vi "playback test.vi"(5 "Rewind":bool, 6 "Record":bool, 7 "Playback":bool, 8 "Taper Limit":dbl=1.0, 9 "Playback allow":bool=TRUE, 10 "Encoder Recording Data":cluster{dbl, u32}[](array[cluster])=[{0.0, 40}, {5.5, 82}, {6.75, 122}, {7.0, 162}, {7.0, 203}, {7.25, 244}, {3.75, 283}, {2.5, 323}, {2.25, 363}, {-0.5, 403}, {-6.75, 444}, {-16.0, 485}, {-28.75, 525}, {-46.0, 565}, {-68.5, 607}, {-94.25, 647}, {-125.25, 689}, {-157.25, 730}, {-189.0, 770}, {-219.75, 811}, {-239.5, 851}, {-265.25, 892}, {-287.0, 932}, {-303.5, 973}, {-312.75, 1014}, {-315.0, 1055}, {-313.5, 1095}, {-306.25, 1136}, {-293.75, 1177}, {-277.0, 1219}, {-254.0, 1261}, {-227.25, 1302}, {-196.0, 1341}, {-158.5, 1382}, {-118.75, 1422}, {-76.75, 1463}, {-36.75, 1503}, {-3.0, 1543}, {26.0, 1583}, {56.5, 1625}, {81.75, 1665}, {100.5, 1706}, {112.5, 1746}, {116.75, 1787}, {116.75, 1828}, {113.0, 1868}, {105.0, 1909}, {92.75, 1949}, {76.25, 1990}, {55.25, 2030}, {29.5, 2071}, {-0.25, 2112}, {-35.25, 2152}, {-74.0, 2193}, {-116.25, 2233}, {-159.0, 2274}, {-202.75, 2314}, {-245.0, 2356}, {-274.5, 2396}, {-310.5, 2436}, {-341.5, 2477}, {-366.25, 2517}, {-383.0, 2558}, {-390.25, 2599}, {-390.75, 2640}, {-387.0, 2681}, {-378.0, 2722}, {-363.0, 2763}, {-343.5, 2804}, {-318.25, 2845}, {-287.0, 2885}, {-248.75, 2926}, {-205.0, 2967}, {-155.75, 3008}, {-102.25, 3049}, {-50.5, 3088}, {1.0, 3130}, {41.25, 3171}, {84.0, 3212}, {122.0, 3253}, {153.75, 3294}, {180.5, 3335}, {200.25, 3375}, {213.5, 3416}, {218.25, 3457}, {218.25, 3496}, {213.5, 3536}, {205.0, 3576}, {192.0, 3617}, {175.0, 3658}, {152.25, 3699}, {125.25, 3740}, {93.5, 3781}, {56.0, 3822}, {13.75, 3863}, {-31.25, 3903}, {-80.25, 3944}, {-130.5, 3986}, {-177.75, 4027}, {-214.25, 4068}, {-253.75, 4108}, {-291.5, 4149}, {-326.0, 4190}, {-356.75, 4231}, {-384.75, 4272}, {-409.5, 4313}, {-431.0, 4353}, {-449.5, 4393}, {-466.0, 4433}, {-479.5, 4474}, {-491.0, 4515}, {-500.0, 4556}, {-506.5, 4597}, {-510.75, 4636}, {-513.0, 4678}, {-513.5, 4718}, {-513.5, 4758}, {-513.5, 4800}, {-513.5, 4840}, {-513.5, 4882}, {-513.5, 4923}, {-513.5, 4964}, {-513.5, 5005}, {-513.5, 5045}, {-513.5, 5085}, {-513.5, 5127}, {-513.5, 5168}, {-513.5, 5211}, {-513.5, 5250}, {-513.5, 5291}, {-513.5, 5331}, {-513.5, 5372}, {-513.5, 5413}, {-513.5, 5454}], 11 "Hardware In":T5={"Motor Selection"="Test motor thing", "EncoderDevRef"={"DevStatus"={"status"=FALSE, "code"=0, "source"=""}, "EncoderIndex"=enum."Enc 0", "CounterIndex"=enum."Invalid", "DistancePerCount"=1.0, "Decoding Type"=enum."4x"}}) -> (0 "Encoder Distance PB":dbl)   [LabVIEW 2017]
uses:
  <vilib>/addons/control/pid/NI_PID_pid.lvlib
  <vilib>/addons/control/pid/pid.llb/PID (DBL).vi
  <vilib>/Rock Robotics/WPI/RobotDrive/WPI_RobotDriveArcadeDrive_Standard(NoSaturation).vi
  <vilib>/Rock Robotics/SystemInterfaces/Encoder/FPGA_EncoderIdx.ctl
  <vilib>/Rock Robotics/WPI/Encoder/WPI_EncoderType.ctl
  <vilib>/Rock Robotics/SystemInterfaces/Counter/FPGA_CounterCtrSystemIndex.ctl
  <vilib>/Rock Robotics/WPI/Encoder/WPI_EncoderDevRef.ctl
panel:
  out "Waveform Chart":cluster{dbl, dbl}(graph)
  in  "Playback PID gains":T6={"proportional gain (Kc)"=0.004, "integral time (Ti, min)"=0.0, "derivative time (Td, min)"=0.0} {"derivative time (Td, min)" format="%.8f"; "integral time (Ti, min)" format="%.8f"; "proportional gain (Kc)" format="%.8f"}
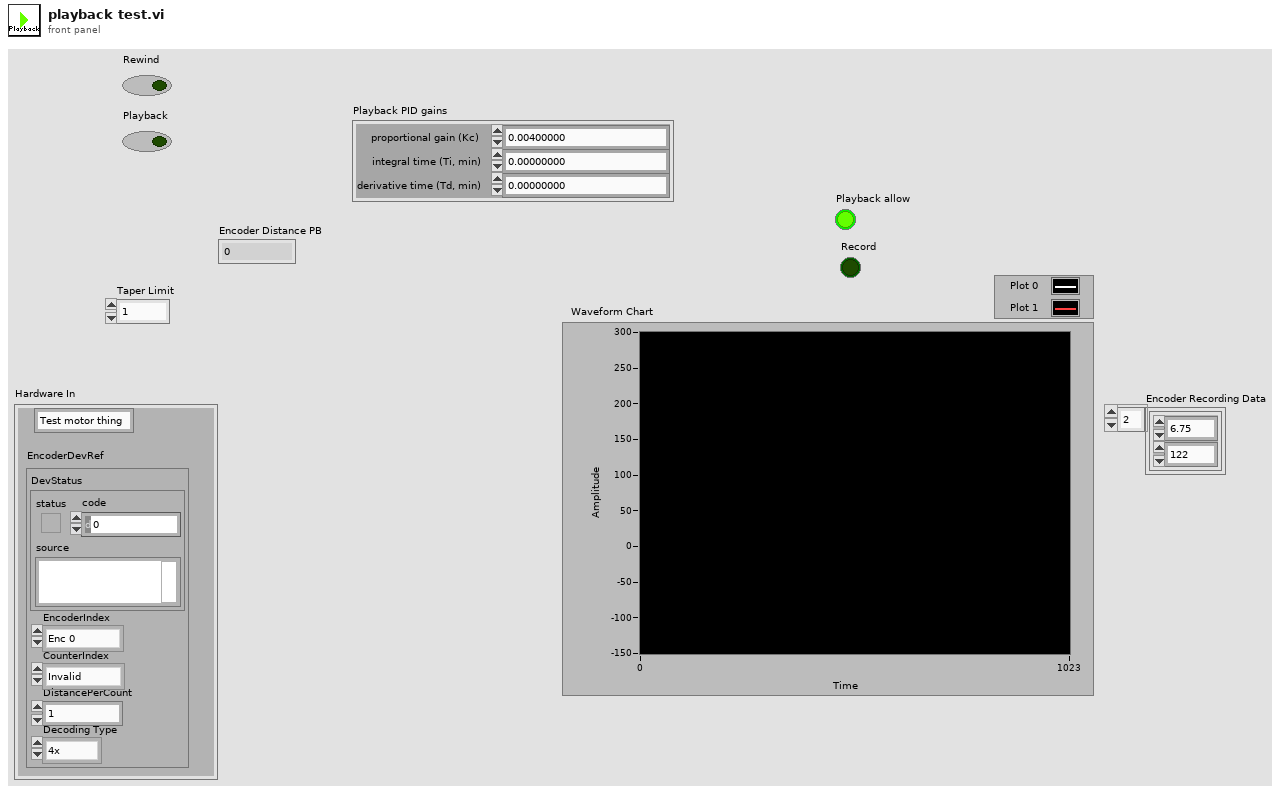
[diagram p1: front panel]
types:
  T1 = typedef "WPI_EncoderDevRef.ctl" = cluster{"DevStatus":errorcluster, "EncoderIndex":T2, "CounterIndex":T3, "DistancePerCount":dbl, "Decoding Type":T4}
  T2 = typedef "FPGA_EncoderIdx.ctl" = enum8{"Enc 0", "Enc 1", "Enc 2", "Enc 3", "Enc 4", "Enc 5", "Enc 6", "Enc 7", "Invalid"}
  T3 = typedef "FPGA_CounterCtrSystemIndex.ctl" = enum8{"Ctr 0", "Ctr 1", "Ctr 2", "Ctr 3", "Ctr 4", "Ctr 5", "Ctr 6", "Ctr 7", "Invalid"}
  T4 = typedef "WPI_EncoderType.ctl" = enum16{"1x", "2x", "4x"}
  T5 = cluster{"Motor Selection":string, "EncoderDevRef":T1}
  T6 = cluster{"proportional gain (Kc)":dbl, "integral time (Ti, min)":dbl, "derivative time (Td, min)":dbl}
  T7 = typedef "WPI_RobotDriveDevRef.ctl" = cluster{"DevStatus":errorcluster, "Motors[]":T8[], "Square Inputs":bool, "Max Output":dbl}
  T8 = typedef "WPI_MotorControlDeviceRef.ctl" = cluster{"DeviceStatus":errorcluster, "Type":T9, "PWM":cluster{"PWM Channel":T10, "DeadBand":T11}, "CAN":cluster{"Device Number":u8, "SetOutput VI Ref":variant, "GetOutput VI Ref":variant, "Enable VI Ref":variant, "Disable VI Ref":variant, "Data":variant}, "Invert":bool, "DIO PWM":cluster{"PWM \"Enable\" Channel":T10, "DIOChannel":T12, "PWM Rate":dbl}}
  T9 = typedef "WPI_MotorControlType.ctl" = enum16{"PWM", "CAN", "DIO PWM"}
  T10 = typedef "FPGA_DIOPWMChannel.ctl" = enum8{"PWM 0", "PWM 1", "PWM 2", "PWM 3", "PWM 4", "PWM 5", "PWM 6", "PWM 7", "PWM 8", "PWM 9", "PWM MXP 0", "PWM MXP 1", "PWM MXP 2", "PWM MXP 3", "PWM MXP 4", "PWM MXP 5", "PWM MXP 6", "PWM MXP 7", "PWM MXP 8", "PWM MXP 9", "Invalid"}
  T11 = typedef "WPI_PWMDeadband.ctl" = cluster{"Name":string, "maxPositivePwm":i32, "minPositivePwm":i32, "centerPwm":i32, "maxNegativePwm":i32, "minNegativePwm":i32, "angularRange":u16}
  T12 = typedef "FPGA_DIOChannel.ctl" = enum8{"DIO 0", "DIO 1", "DIO 2", "DIO 3", "DIO 4", "DIO 5", "DIO 6", "DIO 7", "DIO 8", "DIO 9", "DIO MXP 0", "DIO MXP 1", "DIO MXP 2", "DIO MXP 3", "DIO MXP 4", "DIO MXP 5", "DIO MXP 6", "DIO MXP 7", "DIO MXP 8", "DIO MXP 9", "DIO MXP 10", "DIO MXP 11", "DIO MXP 12", "DIO MXP 13", "DIO MXP 14", "DIO MXP 15", "SPI Port CS1", "SPI Port CS2", "SPI Port CS3", "SPI Port MISO", "SPI Port MOSI", "Invalid"}
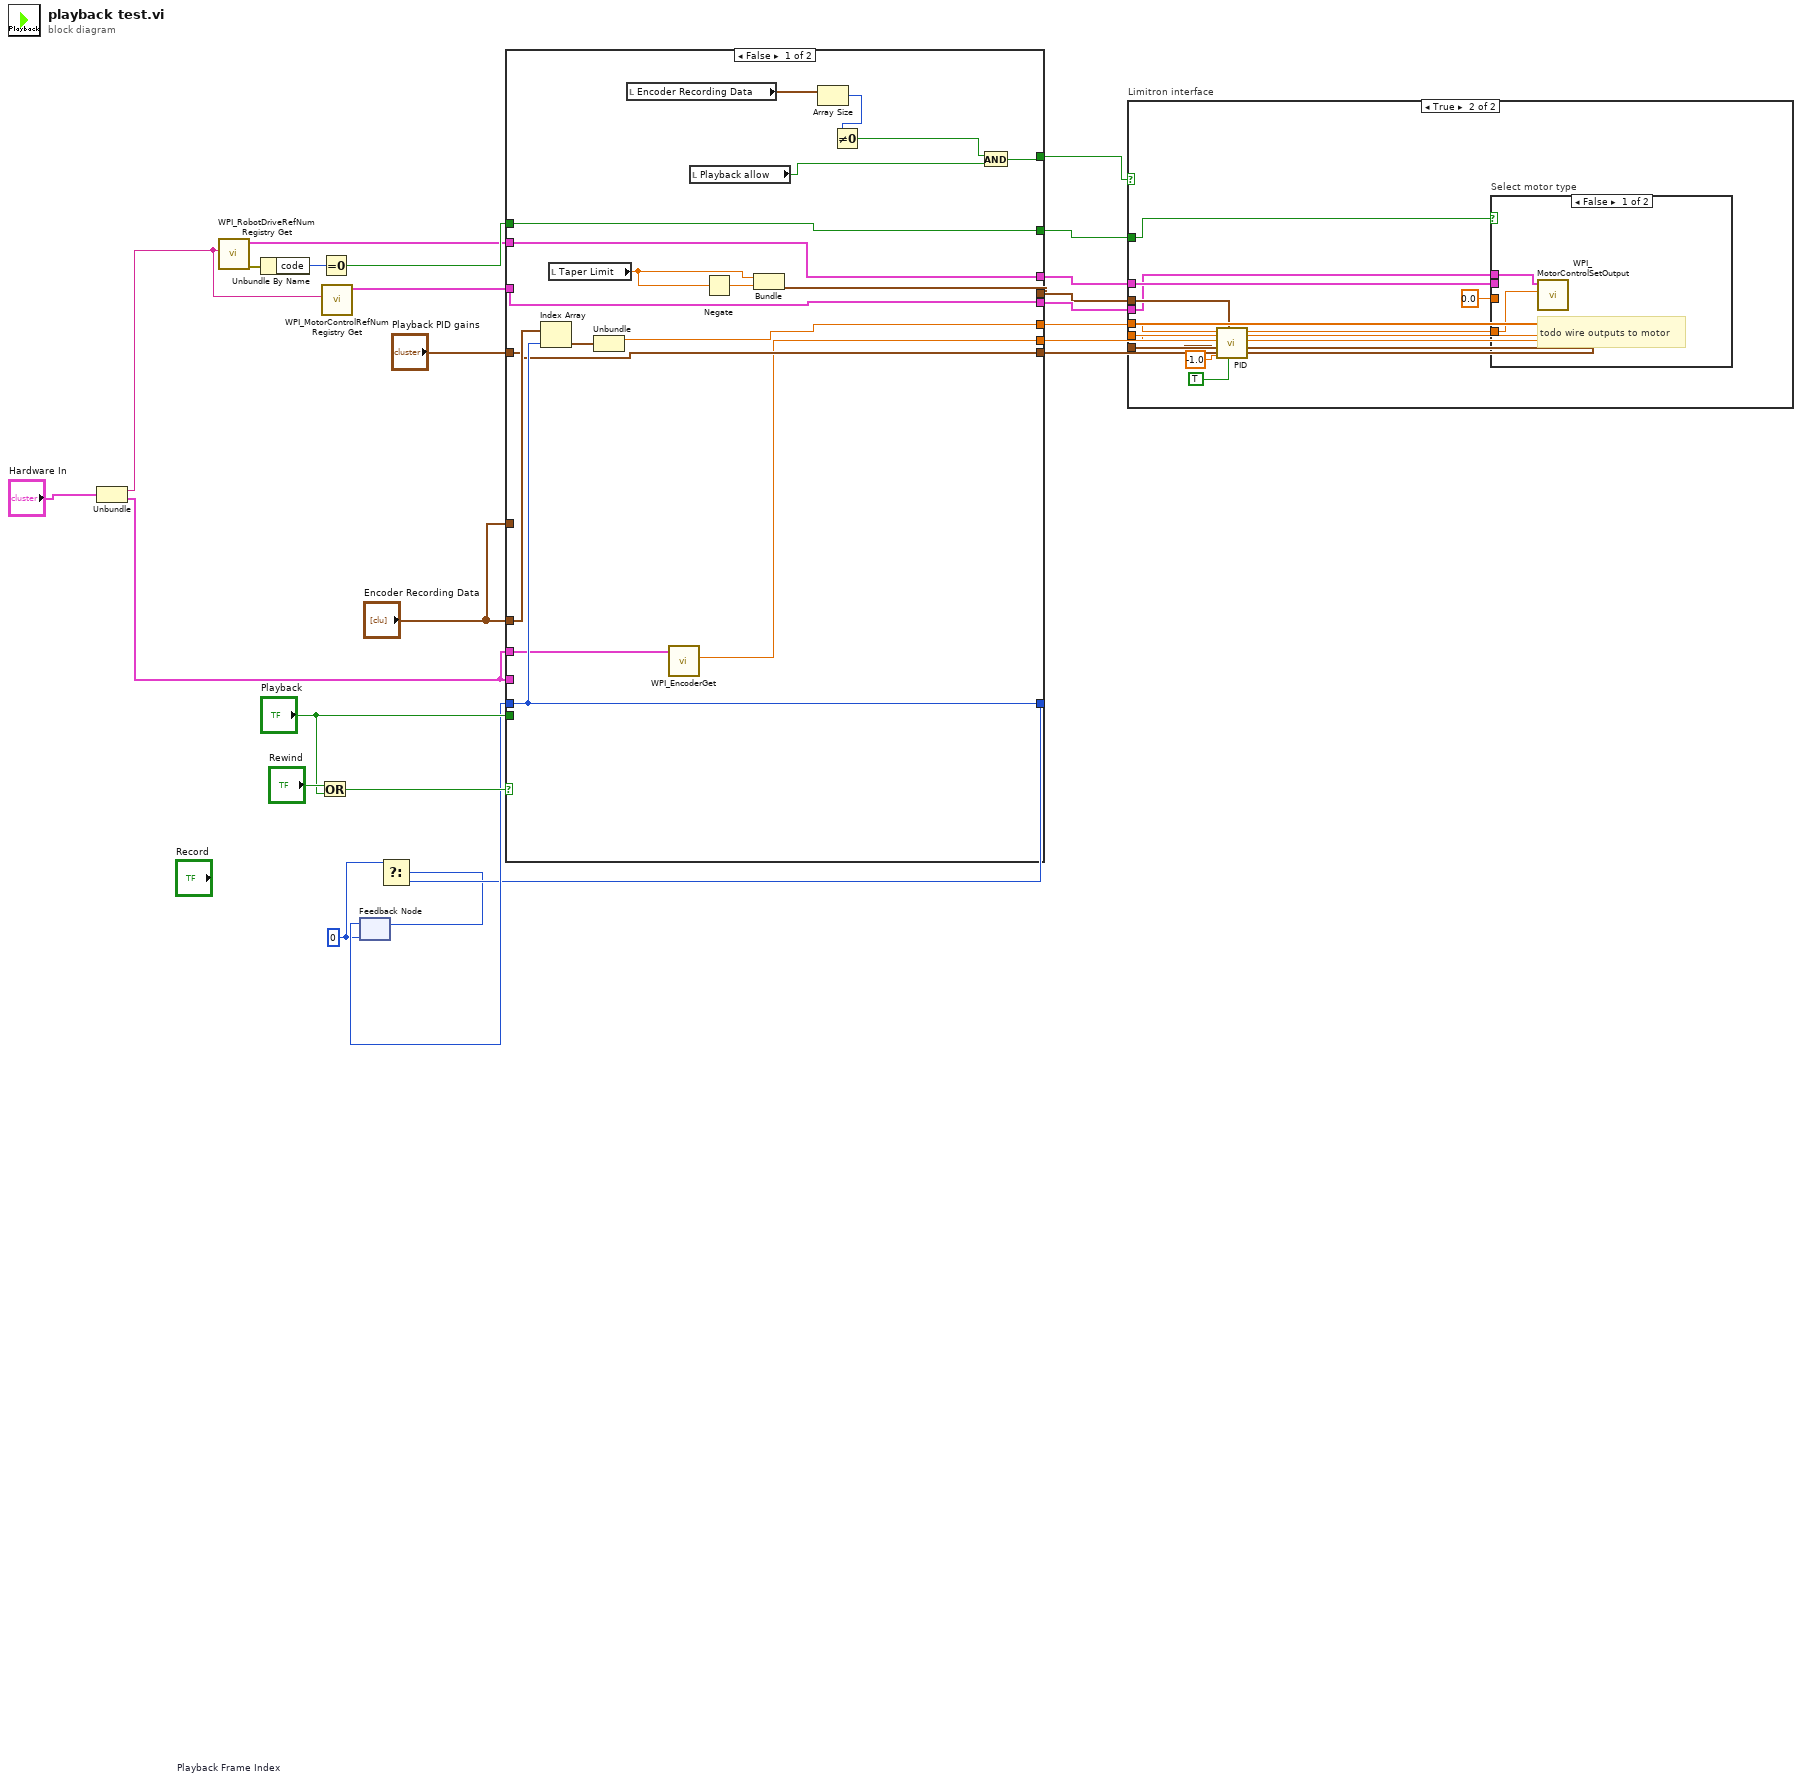
[diagram p0: block diagram]
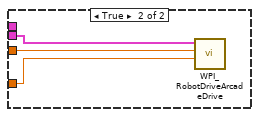
[diagram p3: hidden frame]
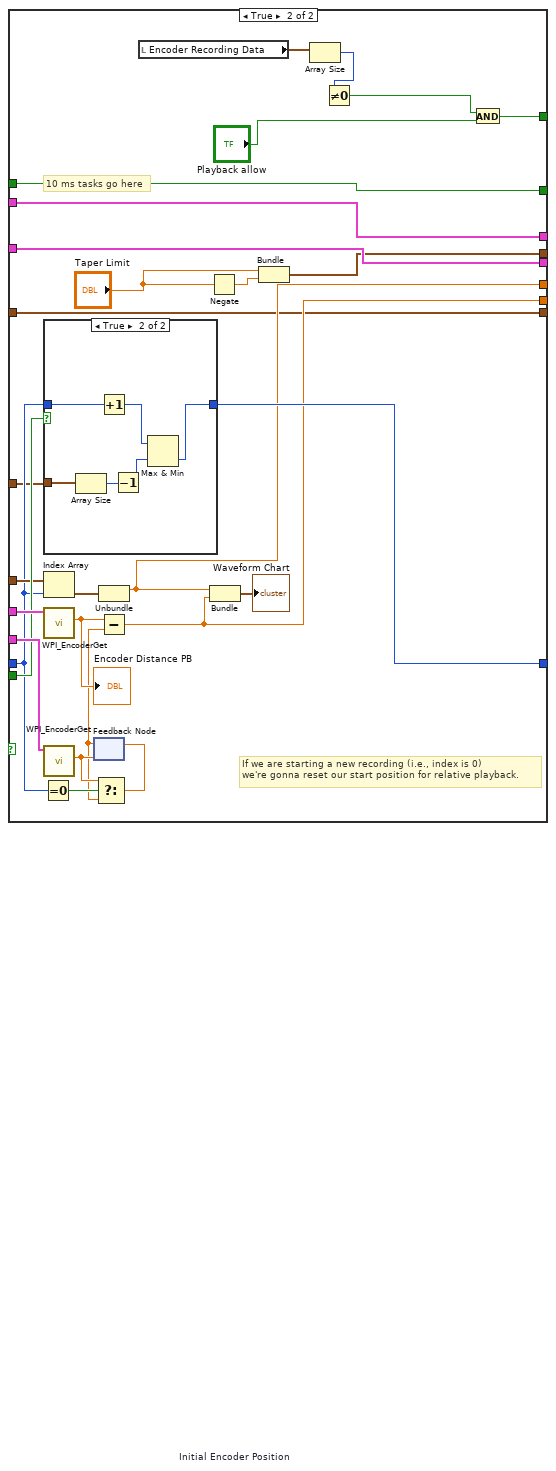
[diagram p4: hidden frame]
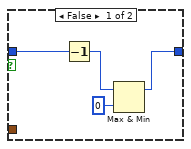
[diagram p5: hidden frame]
diagram:
  w14 = 0 ("index")
  n1 = Unbundle("Hardware In") -> ("Motor Selection"=w10:string, "EncoderDevRef"=w9:T1)
  n2 = call <vilib>:"WPI_RobotDriveRefNum Registry Get.vi"("refnum name"=w10) -> ("error out"=w25:errorcluster, "RobotDriveDevRef"=w23:T7)  [unwired: 1 in, 8 out]
  n3 = Unbundle By Name(w25) -> ("code"=w26:i32)
  n4 = Or(x="Rewind", y="Playback") -> (x .or. y?=w21:bool)
  n5 = Equal To 0?(x=w26) -> (x = 0?=w24:bool)
  n6 = call <vilib>:"WPI_MotorControlRefNum Registry Get.vi"("refnum name"=w10) -> ("MotorControlDevRef"=w19:T8)  [unwired: 9 in, 1 out]
  n7 = feedback #1 "Playback Frame Index"(w14) -> (w18:i32)
  n8 = case shown="False" w21 {
    tunnel: w9 -> [_ w72]
    tunnel: w9 -> [w28 w71]
    tunnel: w24 -> [w39 w56]
    tunnel: w23 -> [w38 w55]
    tunnel: "Playback" -> [_ w70]
    tunnel: w19 -> [w37 w54]
    tunnel: "Encoder Recording Data" -> [w44 w64]
    tunnel: w18 -> [w43 w61]
    tunnel: [w43 w63] -> w15
    tunnel: "Playback PID gains" -> [w35 w50]
    tunnel: "Encoder Recording Data" -> [_ w57]
    tunnel: [w39 w56] -> w8
    tunnel: [w38 w55] -> w7
    tunnel: [w37 w54] -> w6
    tunnel: [w36 w53] -> w5
    tunnel: [w27 w52] -> w4
    tunnel: [w34 w51] -> w3
    tunnel: [w35 w50] -> w2
    tunnel: [w30 w45] -> w1
    frame False {
      n9 = Index Array(array=w44, index=w43) -> (element=w42:cluster{dbl, u32})
      n10 = local read "Taper Limit"() -> (w40:dbl)
      n11 = Unbundle(w42) -> (w36:dbl)  [unwired: 1 out]
      n12 = local read "Encoder Recording Data"() -> (w29:cluster{dbl, u32}[])
      n13 = call <vilib>:"WPI_EncoderGet.vi"("EncoderDevRef"=w28) -> ("Distance"=w27:dbl)  [unwired: 5 in, 5 out]
      n14 = local read "Playback allow"() -> (w31:bool)
      n15 = Negate(x=w40) -> (-x=w41:dbl)
      n16 = Bundle("Taper Limit"=w40, w41) -> (w34:cluster{"Taper Limit":dbl, dbl})  [unwired: 1 in]
      n17 = Array Size(array=w29) -> (size(s)=w33:i32)
      n18 = Not Equal To 0?(x=w33) -> (x != 0?=w32:bool)
      n19 = And(x=w32, y=w31) -> (x .and. y?=w30:bool)
    }
    frame True {
      # "If we are starting a new recording (i.e., index is 0)\nwe're gonna reset our start position for relative playback."
      # "10 ms tasks go here"
      n20 = Equal To 0?(x=w61) -> (x = 0?=w62:bool)
      n21 = case shown="True" w70 {
        tunnel: [w73 w80] -> w63
        tunnel: w61 -> [w76 w82]
        tunnel: w57 -> [_ w79]
        frame False {
          n22 = Decrement(x=w76) -> (x-1=w74:i32)
          n23 = Max & Min(x=w74, y=0) -> (max(x,y)=w73:i32)  [unwired: 1 out]
        }
        frame True {
          n24 = Array Size(array=w79) -> (size(s)=w78:i32)
          n25 = Increment(x=w82) -> (x+1=w81:i32)
          n26 = Decrement(x=w78) -> (x-1=w77:i32)
          n27 = Max & Min(x=w81, y=w77) -> (min(x,y)=w80:i32)  [unwired: 1 out]
        }
      }
      n28 = Index Array(array=w64, index=w61) -> (element=w65:cluster{dbl, u32})
      n29 = call <vilib>:"WPI_EncoderGet.vi"("EncoderDevRef"=w71) -> ("Distance"=w69:dbl)  [unwired: 5 in, 5 out]
      "Encoder Distance PB" <- w69
      n30 = call <vilib>:"WPI_EncoderGet.vi"("EncoderDevRef"=w72) -> ("Distance"=w60:dbl)  [unwired: 5 in, 5 out]
      n31 = feedback #2 "Initial Encoder Position"(w60) -> (w58:dbl)
      n32 = Select(t=w60, s=w62, f=w58) -> (s? t:f=w59:dbl)
      n33 = feedback-in #2(w59) -> ()
      n34 = Unbundle(w65) -> (w53:dbl)  [unwired: 1 out]
      n35 = Subtract(x=w69, y=w58) -> (x-y=w52:dbl)
      n36 = local read "Encoder Recording Data"() -> (w48:cluster{dbl, u32}[])
      n37 = Negate(x="Taper Limit") -> (-x=w67:dbl)
      n38 = Bundle(w53, w52) -> (→"Waveform Chart":cluster{dbl, dbl})  [unwired: 1 in]
      n39 = Bundle("Taper Limit"="Taper Limit", w67) -> (w51:cluster{"Taper Limit":dbl, dbl})  [unwired: 1 in]
      n40 = Array Size(array=w48) -> (size(s)=w49:i32)
      n41 = Not Equal To 0?(x=w49) -> (x != 0?=w46:bool)
      n42 = And(x=w46, y="Playback allow") -> (x .and. y?=w45:bool)
    }
  }
  n43 = Select(t=w14, f=w15) -> (s=w16:bool, s? t:f=w13:i32)
  n44 = feedback-in #1(w13) -> ()
  n45 = case "Limitron interface" shown="True" w1 {
    tunnel: w2 -> [_ w93]
    tunnel: w4 -> [_ w90]
    tunnel: w5 -> [_ w89]
    tunnel: w6 -> [_ w84]
    tunnel: w8 -> [_ w85]
    tunnel: w7 -> [_ w87]
    tunnel: w3 -> [_ w86]
    frame False {
    }
    frame True {
      n46 = call-poly <vilib>:"PID.vi"("reinitialize? (F)"=TRUE, "output range"=w86, "dt (s)"=-1.0, "PID gains"=w93, "process variable"=w90, "setpoint"=w89) -> ("output"=w88:dbl)  [unwired: 4 in, 1 out]
      n47 = case "Select motor type" shown="False" w85 {
        tunnel: 0.0 ("output") -> [_ w98]
        tunnel: w88 -> [w95 w97]
        tunnel: w87 -> [_ w96]
        tunnel: w84 -> [w94 _]
        frame False {
          # "todo wire outputs to motor"
          n48 = call <vilib>:"WPI_MotorControlSetOutput.vi"("Output"=w95, "MotorControlDevRef"=w94) -> ()  [unwired: 7 in, 3 out]
        }
        frame True {
          n49 = call-poly <vilib>:"WPI_RobotDriveArcadeDrive.vi"("Y axis value"=w97, "X axis value"=w98, "RobotDriveDevRef"=w96) -> ()  [unwired: 6 in, 3 out]
        }
      }
    }
  }
